vi "configure.vi"(8 "error in (no error)":errorcluster, 11 "GenericPlugin in":refnum<class "TrajectoryMG100122AODFrameScan.lvclass">) -> (0 "error out":errorcluster, 3 "GenericPlugin out":refnum<class "TrajectoryMG100122AODFrameScan.lvclass">)   [LabVIEW 2010, in "TrajectoryMG100122AODFrameScan.lvclass"]
doc: "The dynamic dispatch version of this VI loads and displays the configuration file associated with the plug-in object. The user modify and save the configuration data."
uses:
  TrajectoryMG100122AODFrameScan.lvclass
  common/xcontrols/XComponentSpecification/XComponentSpecification/XComponentSpecification.xctl
  TrajectoryMG100122AODFrameScan.lvclass/TrajectoryMG100122AODFrameScan.ctl
  common/classes/GenericComponent/GenericComponent/GenericComponent.lvclass
panel:
  in  "FOVy":dbl[unit]
  in  "FOVx":dbl[unit]
  in  "FPGA Wrapper path":T1(xcontrol)
  in  "cancel":bool
  in  "save":bool
  out "Configuration name":string
  # "Configure TrajectoryAODFrameScan"
  # "Note\nMeasure the Field Of View at zoom 1x and use the stage to measure left-to-right and top-to bottom."
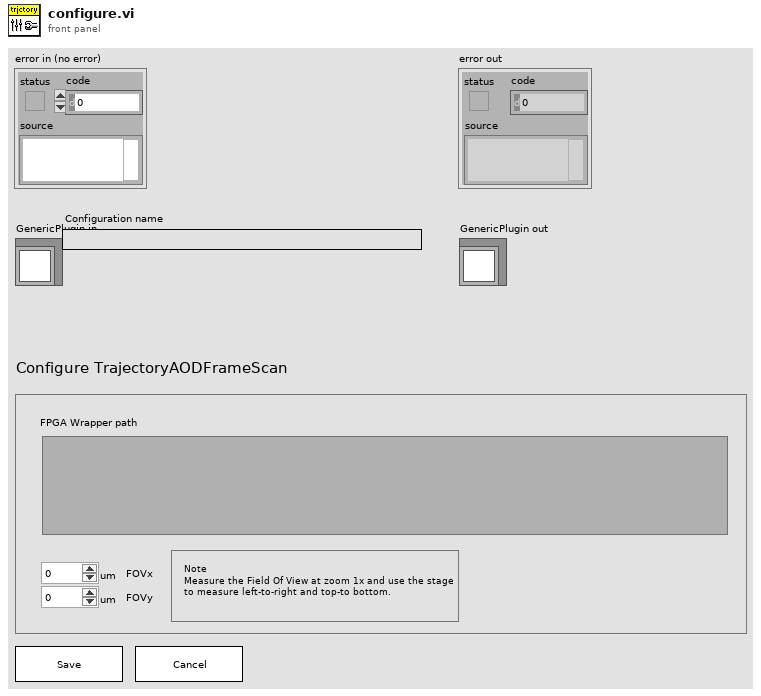
[diagram p1: front panel]
types:
  T1 = cluster{"class path":string, "configuration":string, "label":string, "settings name":string}
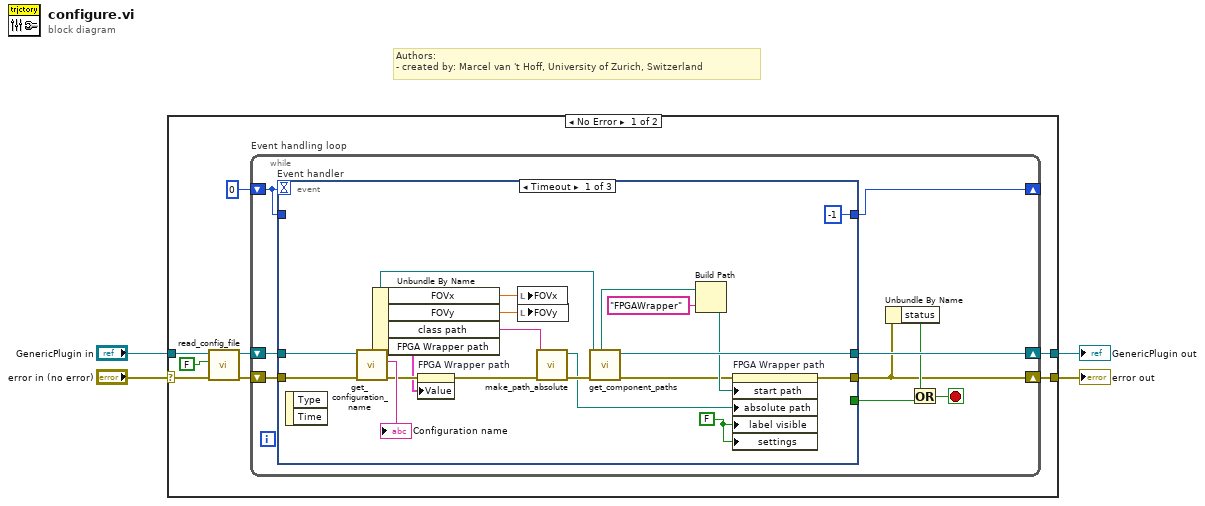
[diagram p0: block diagram]
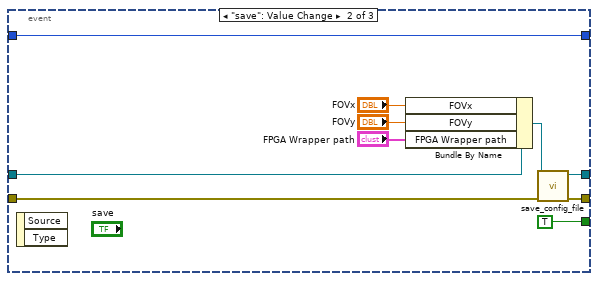
[diagram p2: hidden frame]
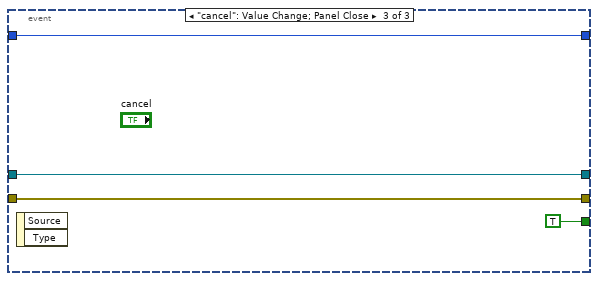
[diagram p3: hidden frame]
diagram:
  # "Authors: \n- created by: Marcel van 't Hoff, University of Zurich, Switzerland"
  n1 = case shown="No Error" "error in (no error)" {
    selector: "error in (no error)" -> [w9 w57]
    tunnel: [w11 w57] -> w4
    tunnel: [w10 w56] -> w3
    tunnel: "GenericPlugin in" -> [w8 w56]
    frame No Error {
      n2 = call-dynamic "read_config_file.vi"("error in (no error)"=w9, "force load?"=FALSE, "GenericPlugin in"=w8) -> ("error out"=w5:errorcluster, "GenericPlugin out"=w7:refnum<class "TrajectoryMG100122AODFrameScan.lvclass">)  [unwired: 7 out]
      n3 = while "Event handling loop" {
        shift-right: [w19] -> _
        shift-left: 0 -> [w20]
        shift-right: [w15] -> w11
        shift-left: w5 -> [w21]
        shift-right: [w17] -> w10
        shift-left: w7 -> [w18]
        stop <- w14 stop-if-true
        n4 = event "Event handler" shown="[0] Timeout" {
          selector: _ -> [_ _ _]
          dyn-events: _ -> [_ _ _]
          timeout: w20 -> [_ _ _]
          tunnel: w21 -> [w40 w44 w54]
          tunnel: [-1 w51 w55] -> w19
          tunnel: w20 -> [_ w51 w55]
          tunnel: [w30 w50 w54] -> w15
          tunnel: [_ TRUE TRUE] -> w13
          tunnel: w18 -> [w39 w47 w52]
          tunnel: [w36 w49 w52] -> w17
          event Timeout {
            w29 = FALSE
            n5 = event-data() -> ()  [unwired: 3 out]
            n6 = call "get_configuration_name.vi"("error in (no error)"=w40, "GenericPlugin.lvclass in"=w39) -> ("error out"=w26:errorcluster, "configuration name"=→"Configuration name":string, "GenericPlugin.lvclass out"=w37:refnum<class "TrajectoryMG100122AODFrameScan.lvclass">)  [unwired: 7 in]
            n7 = Unbundle By Name(w37) -> ("FOVx"=w23:dbl[unit], "FOVy"=w22:dbl[unit], "class path"=w28:string, "FPGA Wrapper path"=w24:T1)
            n8 = property on="FPGA Wrapper path" class="XComponentSpecification (strict"(error in=w26, "Value"=w24) -> (error out=w25:errorcluster)  [unwired: 1 in, 1 out]
            n9 = local write "FOVx"(w23) -> ()
            n10 = local write "FOVy"(w22) -> ()
            n11 = call "make_path_absolute.vi"("error in (no error)"=w25, "relative path"=w28) -> ("error out"=w35:errorcluster, "absolute path"=w27:path)  [unwired: 8 in]
            n12 = call-dynamic "get_component_paths.vi"("error in (no error)"=w35, "GenericComponent in"=w37) -> ("error out"=w31:errorcluster, "GenericComponent out"=w36:refnum<class "TrajectoryMG100122AODFrameScan.lvclass">, "components directory"=w33:path)  [unwired: 4 in, 3 out]
            n13 = Build Path(base path=w33, name or relative path="FPGAWrapper") -> (appended path=w32:path)
            n14 = property on="FPGA Wrapper path" class="XComponentSpecification (strict"(error in=w31, "start path"=w32, "absolute path"=w27, "label visible"=w29, "settings"=w29) -> (error out=w30:errorcluster)  [unwired: 1 in, 1 out]
          }
          event "save": Value Change {
            n15 = event-data() -> ()  [unwired: 3 out]
            n16 = Bundle By Name(cluster=w47, "FOVx"="FOVx", "FOVy"="FOVy", "FPGA Wrapper path"="FPGA Wrapper path") -> (w46:refnum<class "TrajectoryMG100122AODFrameScan.lvclass">)
            n17 = call-dynamic "save_config_file.vi"("error in (no error)"=w44, "GenericPlugin in"=w46) -> ("error out"=w50:errorcluster, "GenericPlugin out"=w49:refnum<class "TrajectoryMG100122AODFrameScan.lvclass">)  [unwired: 2 in, 6 out]
          }
          event "cancel": Value Change; Panel Close {
            n18 = event-data() -> ()  [unwired: 3 out]
          }
        }
        n19 = Unbundle By Name(w15) -> ("status"=w16:bool)
        n20 = Or(x=w16, y=w13) -> (x .or. y?=w14:bool)
      }
    }
    frame Error {
    }
  }
  "error out" <- w4
  "GenericPlugin out" <- w3
